vi "Generate step array.vi"(4 "Step":dbl, 6 "Add step back":bool, 7 "Increment mode":T1, 9 "Number of steps":i32, 10 "End":dbl, 11 "Start":dbl) -> (3 "Steps":dbl[](array[numeric]))   [LabVIEW 2024]
uses:
  Increment mode.ctl
panel:
  out "Steps graph":dbl[](graph)
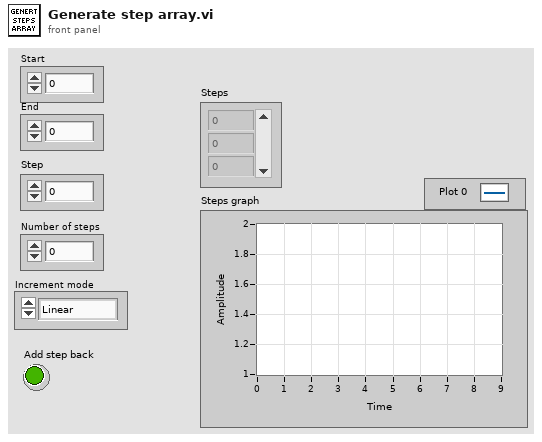
[diagram p1: front panel]
types:
  T1 = typedef "Increment mode.ctl" = enum16{"Linear", "Square root", "Square", "Log", "Exponent"}
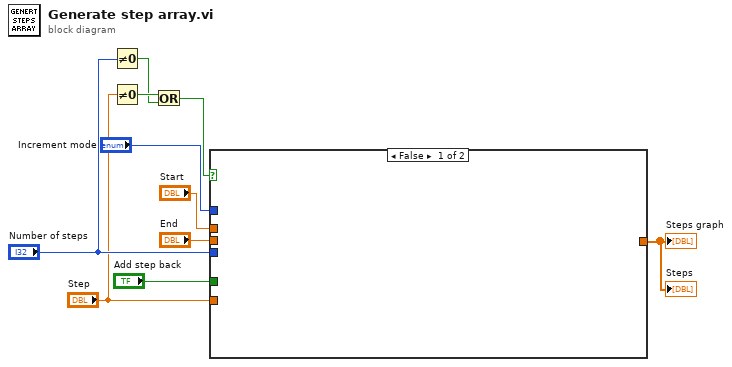
[diagram p0: block diagram]
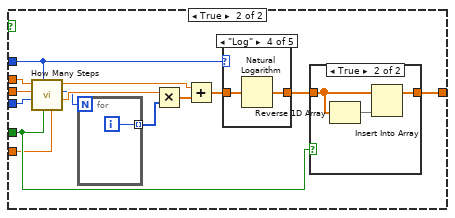
[diagram p2: hidden frame]
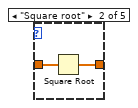
[diagram p5: hidden frame]
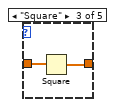
[diagram p6: hidden frame]
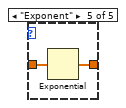
[diagram p7: hidden frame]
diagram:
  n1 = Not Equal To 0?(x="Number of steps") -> (x != 0?=w2:bool)
  n2 = Not Equal To 0?(x="Step") -> (x != 0?=w3:bool)
  n3 = Or(x=w3, y=w2) -> (x .or. y?=w1:bool)
  n4 = case shown="False" w1 {
    tunnel: [_ w23] -> w10
    tunnel: "Start" -> [_ w16]
    tunnel: "End" -> [_ w15]
    tunnel: "Add step back" -> [_ w14]
    tunnel: "Increment mode" -> [_ w13]
    tunnel: "Number of steps" -> [_ w12]
    tunnel: "Step" -> [_ w11]
    frame False {
    }
    frame True {
      n5 = call "How Many Steps.vi"("Step"=w11, "Add step back"=w14, "Increment mode"=w13, "Number of steps"=w12, "End"=w15, "Start"=w16) -> ("Step out"=w19:dbl, "Number of steps out"=w18:i32, "Start out"=w17:dbl)  [unwired: 3 in]
      n6 = for {
        N: w18 -> [_]
        tunnel: [w38] -> w21 mode=indexing
        i -> [w38]
      }
      n7 = Multiply(x=w19, y=w21) -> (x*y=w22:dbl[])
      n8 = Add(x=w17, y=w22) -> (x+y=w20:dbl[])
      n9 = case shown="\"Log\"" w13 {
        tunnel: w20 -> [w29 w31 w33 w35 w37]
        tunnel: [w29 w30 w32 w34 w36] -> w24
        frame "Linear", Default {
        }
        frame "Square root" {
          n10 = Square Root(x=w31) -> (sqrt(x)=w30:dbl[])
        }
        frame "Square" {
          n11 = Square(x=w33) -> (x^2=w32:dbl[])
        }
        frame "Log" {
          n12 = Natural Logarithm(1:w35) -> (0:w34:dbl[])
        }
        frame "Exponent" {
          n13 = Exponential(1:w37) -> (0:w36:dbl[])
        }
      }
      n14 = case shown="True" w14 {
        tunnel: w24 -> [w25 w28]
        tunnel: [w25 w26] -> w23
        frame False {
        }
        frame True {
          n15 = Reverse 1D Array(array=w28) -> (reversed array=w27:dbl[])
          n16 = Insert Into Array(array=w28, new element=w27) -> (w26:dbl[])  [unwired: 1 in]
        }
      }
    }
  }
  "Steps" <- w10
  "Steps graph" <- w10
